vi "Init.vi"(11 "error in (no error)":errorcluster) -> (4 "FPGA API out":refnum<class "FPGA API.lvclass">, 15 "error out":errorcluster)   [LabVIEW 2019, in "FPGA API.lvclass"]
uses:
  FPGA API.lvclass
  FPGA/TypeDef/DO index.ctl
  FPGA Ref.ctl
  FPGA API.lvclass/FPGA API.ctl
  <vilib>/FPGAPlugInAG/cRIO-9035/niLvFpga_Open_cRIO-9035.vi
  <vilib>/rvi/interface/common/dynamic/niFpgaDynamicAddResources.vi
  <vilib>/rvi/interface/common/niFpgaWaitOnOcc.vi
  <vilib>/Utility/error.llb/Error Cluster From Error Code.vi
  <vilib>/rvi/interface/nirviOpenFPGA/nirviOpenFPGA.xnode
  FPGA Bitfiles/hydrort_FPGATarget_MAINFPGAV2_ZQcTIcjWSFE.lvbitx
  <vilib>/rvi/interface/nirviMethod/nirviMethod.xnode
  <vilib>/rvi/errors/niLvFpgaMergeErrorWithErrorCode.vi
  <vilib>/FPGAPlugInAG/Dynamic/niLvFpga_ConfigureFifo_Dynamic.vi
  <vilib>/FPGAPlugInAG/Dynamic/niLvFpga_StartFifo_Dynamic.vi
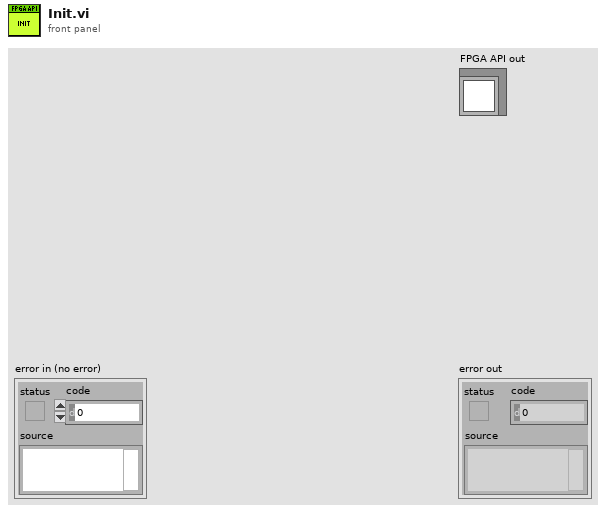
[diagram p1: front panel]
types:
  T1 = typedef "DO index.ctl" = u8
  T2 = typedef "FPGA API.lvclass/FPGA Ref.ctl" = refnum<k20>
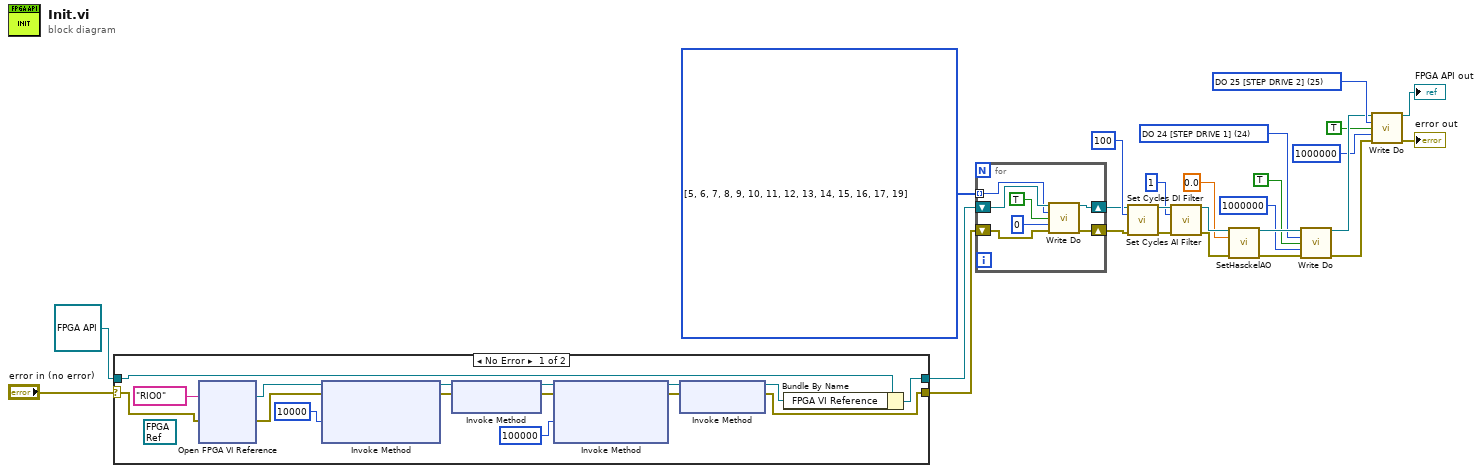
[diagram p0: block diagram]
diagram:
  w8 = T1 25 items=["DO 0 [KP1 [DO 0]]", "DO 1 [ON KP2 [DO 1]]", "DO 2 [ON KP3 [DO 2]]", "DO 3 [WATER Y18.1 [DO3]]", "DO 4 [WATER Y18.2 [DO4]]", "DO 5 [KP6 Y29.1 33.7]", "DO 6 [KP7 Y29.2 33.8]", "DO 7 [KP8 Y29.3 33.9]", "DO 8 [KP9 Y29.4  33.12]", "DO 9 [KP10 Y29.5 33.1]", "DO 10 [KP11 Y29.6 33.2]", "DO 11 [KP12 Y29.7  33.13]", "DO 12 [KP13 Y29.8  33.11]", "DO 13 [KP14 Y29.9 33.10]", "DO 14 [KP15 Y29.10  33.6]", "DO 15 [KP16 Y29.11  33.5]", "DO 16 [KP17 Y29.12  33.4]", "DO 17 [KP18 Y29.13 33.3]", "DO 18 [AIR KP19]", "DO 19 [STEP DRIVE EN KP20]", "DO 20 [KP21 Y44.1 OPEN]", "DO 21 [ KP22 Y44.1 CLOSE]", "DO 22 [ KP23 Y44.2 OPEN]", "DO 23", "DO 24 [STEP DRIVE 1]", "DO 25 [STEP DRIVE 2]"] ("#DO")
  w11 = T1 24 items=["DO 0 [KP1 [DO 0]]", "DO 1 [ON KP2 [DO 1]]", "DO 2 [ON KP3 [DO 2]]", "DO 3 [WATER Y18.1 [DO3]]", "DO 4 [WATER Y18.2 [DO4]]", "DO 5 [KP6 Y29.1 33.7]", "DO 6 [KP7 Y29.2 33.8]", "DO 7 [KP8 Y29.3 33.9]", "DO 8 [KP9 Y29.4  33.12]", "DO 9 [KP10 Y29.5 33.1]", "DO 10 [KP11 Y29.6 33.2]", "DO 11 [KP12 Y29.7  33.13]", "DO 12 [KP13 Y29.8  33.11]", "DO 13 [KP14 Y29.9 33.10]", "DO 14 [KP15 Y29.10  33.6]", "DO 15 [KP16 Y29.11  33.5]", "DO 16 [KP17 Y29.12  33.4]", "DO 17 [KP18 Y29.13 33.3]", "DO 18 [AIR KP19]", "DO 19 [STEP DRIVE EN KP20]", "DO 20 [KP21 Y44.1 OPEN]", "DO 21 [ KP22 Y44.1 CLOSE]", "DO 22 [ KP23 Y44.2 OPEN]", "DO 23", "DO 24 [STEP DRIVE 1]", "DO 25 [STEP DRIVE 2]"] ("#DO")
  w19 = T1[] [5, 6, 7, 8, 9, 10, 11, 12, 13, 14, 15, 16, 17, 19] items=["DO 0 [KP1 [DO 0]]", "DO 1 [ON KP2 [DO 1]]", "DO 2 [ON KP3 [DO 2]]", "DO 3 [WATER Y18.1 [DO3]]", "DO 4 [WATER Y18.2 [DO4]]", "DO 5 [KP6 Y29.1 33.7]", "DO 6 [KP7 Y29.2 33.8]", "DO 7 [KP8 Y29.3 33.9]", "DO 8 [KP9 Y29.4  33.12]", "DO 9 [KP10 Y29.5 33.1]", "DO 10 [KP11 Y29.6 33.2]", "DO 11 [KP12 Y29.7  33.13]", "DO 12 [KP13 Y29.8  33.11]", "DO 13 [KP14 Y29.9 33.10]", "DO 14 [KP15 Y29.10  33.6]", "DO 15 [KP16 Y29.11  33.5]", "DO 16 [KP17 Y29.12  33.4]", "DO 17 [KP18 Y29.13 33.3]", "DO 18 [AIR KP19]", "DO 19 [STEP DRIVE EN KP20]", "DO 20 [KP21 Y44.1 OPEN]", "DO 21 [ KP22 Y44.1 CLOSE]", "DO 22 [ KP23 Y44.2 OPEN]", "DO 23", "DO 24 [STEP DRIVE 1]", "DO 25 [STEP DRIVE 2]"] ("#DO")
  n1 = case shown="No Error" "error in (no error)" {
    selector: "error in (no error)" -> [w36 w44]
    tunnel: [w27 w44] -> w20
    tunnel: [w34 w43] -> w23
    tunnel: refnum<class "FPGA API.lvclass"> refnum ("FPGA API in") -> [w42 w43]
    frame No Error {
      (unwired) T2 refnum ("FPGA VI Reference")
      n2 = xnode "Open FPGA VI Reference"("error in"=w36, "resource name"=tag "RIO0") -> ("FPGA VI Reference Out"=w41:refnum<k20>, "error out"=w37:errorcluster)
      n3 = xnode "Invoke Method"("FPGA VI Reference In"=w41, "error in"=w37, "Requested Depth"=u32 10000) -> ("FPGA VI Reference Out"=w39:refnum<k20>, "error out"=w38:errorcluster)  [unwired: 1 out]
      n4 = xnode "Invoke Method"("FPGA VI Reference In"=w39, "error in"=w38) -> ("FPGA VI Reference Out"=w30:refnum<k20>, "error out"=w29:errorcluster)
      n5 = xnode "Invoke Method"("FPGA VI Reference In"=w30, "error in"=w29, "Requested Depth"=u32 100000) -> ("FPGA VI Reference Out"=w33:refnum<k20>, "error out"=w32:errorcluster)  [unwired: 1 out]
      n6 = xnode "Invoke Method"("FPGA VI Reference In"=w33, "error in"=w32) -> ("FPGA VI Reference Out"=w28:refnum<k20>, "error out"=w27:errorcluster)
      n7 = Bundle By Name(cluster=w42, "FPGA VI Reference"=w28) -> (w34:refnum<class "FPGA API.lvclass">)
    }
    frame Error {
    }
  }
  n8 = for {
    tunnel: w19 -> [w47] mode=indexing
    shift-right: [w50] -> w22
    shift-left: w23 -> [w51]
    shift-right: [w49] -> w21
    shift-left: w20 -> [w48]
    n9 = call "Write Do.vi"("FPGA API in"=w51, "#DO"=w47, "value"=TRUE, "Time uSec"=u32 0, "error in (no error)"=w48) -> ("FPGA API out"=w50:refnum<class "FPGA API.lvclass">, "error out"=w49:errorcluster)  [unwired: 9 in]
  }
  n10 = call "Set Cycles DI Filter.vi"("FPGA API in"=w22, "Cycles to Filter"=u16 100, "error in (no error)"=w21) -> ("FPGA API out"=w18:refnum<class "FPGA API.lvclass">, "error out"=w17:errorcluster)  [unwired: 11 in]
  n11 = call "Set Cycles AI Filter.vi"("FPGA API in"=w18, "Cycles to Filter"=u16 1, "error in (no error)"=w17) -> ("FPGA API out"=w15:refnum<class "FPGA API.lvclass">, "error out"=w14:errorcluster)  [unwired: 11 in]
  n12 = call "SetHasckelAO.vi"("FPGA API in"=w15, "Haskel in"=0.0, "error in (no error)"=w14) -> ("FPGA API out"=w12:refnum<class "FPGA API.lvclass">, "error out"=w4:errorcluster)  [unwired: 11 in]
  n13 = call "Write Do.vi"("FPGA API in"=w12, "#DO"=w11, "value"=TRUE, "Time uSec"=u32 1000000, "error in (no error)"=w4) -> ("FPGA API out"=w7:refnum<class "FPGA API.lvclass">, "error out"=w3:errorcluster)  [unwired: 9 in]
  n14 = call "Write Do.vi"("FPGA API in"=w7, "#DO"=w8, "value"=TRUE, "Time uSec"=u32 1000000, "error in (no error)"=w3) -> ("FPGA API out"=→"FPGA API out":refnum<class "FPGA API.lvclass">, "error out"=→"error out":errorcluster)  [unwired: 9 in]
